vi "Main.vi"() -> ()   [LabVIEW 2026]
doc: "VI TIMESTAMP — DOCUMENTATION\n============================\nInstitut Fresnel | USB-6353 | CTR3 | PFI7 | 100 MHz | LabVIEW 2025\n\n\nOBJECTIF\n--------\nEnregistrer le timestamp absolu de chaque trigger caméra avec une\nprécision hardware de 10 ns. Résultat écrit dans un fichier CSV,\nécrasé à chaque nouvelle acquisition.\n\n\nPRINCIPE\n--------\nCTR3 compte les ticks de l'horloge interne 100 MHz. Le signal trigger\n(P0.4, rebouclé sur PFI7) est l'horloge d'échantillonnage : à chaque\nflanc montant, CTR3 capture la valeur courante du compteur.\n\n T_absolu = T0 + (ticks + offset_rollover) / 100 000 000\n\nT0 = heure système au démarrage (Get Date/Time In Seconds).\noffset_rollover = compensation du débordement 32 bits (rollover ~42.9 s).\n\n\nMACHINE À ÉTATS\n---------------\nIDLE ? INIT ? START ? RUNNING ? WRITE ? STOP ? IDLE\n\n IDLE : attente bouton Start, lecture N (nb frames)\n INIT : création tâche CTR3, config timing PFI7, ouverture CSV, T0\n START : DAQmx Start Task — doit précéder les tâches DO/AO du VI principal\n RUNNING : DAQmx Read non-bloquant (timeout 0.01 s) — boucle sur lui-même\n WRITE : calcul timestamp, gestion rollover, écriture ligne CSV\n STOP : Stop Task, Clear Task, Close File, reset SR\n\n\nGESTION ROLLOVER (dans WRITE)\n------------------------------\n Si ticks < ticks_prev ? offset += 4 294 967 296\n ticks_prev ? ticks (valeur brute, sans offset)\n\n\nSHIFT REGISTERS\n---------------\n état Enum État courant\n task ref DAQmx Task Référence CTR3\n file ref File Refnum Fichier CSV ouvert\n T0 Timestamp Heure au Start\n ticks DBL Valeur DAQmx Read\n ticks_prev DBL (init 0) Ticks de la frame précédente\n offset DBL (init 0) Cumul rollovers × 2^32\n frame_i I32 (init 0) Index frame courante\n\n\nFORMAT CSV\n----------\n frame_index I32 Index frame (0-indexé)\n timestamp_iso String Ex : 2026-03-09T11:13:54.223 (ISO 8601)\n timestamp_unix DBL Ex : 3855896034.224 (secondes depuis 01/01/1904)\n\nConversion Python :\n df['datetime'] = pd.to_datetime(df['timestamp_unix'] - 2082844800, unit='s')\n\n\nVALIDATION\n----------\n 20.9 Hz jitter 358 µs (vient du générateur NI-MAX, pas du VI) ?\n 0.1 Hz 2 rollovers détectés et compensés, monotonie OK ?"
uses:
  controls/State.ctl
  <vilib>/DAQmx/read.llb/DAQmx Read (Counter DBL 1Chan 1Samp).vi
  <vilib>/DAQmx/create/channels.llb/DAQmx Create Channel (CI-Count Edges).vi
  <vilib>/DAQmx/configure/timing.llb/DAQmx Timing (Sample Clock).vi
  <vilib>/DAQmx/miscellaneous.llb/DAQmx Fill In Error Info.vi
  <vilib>/Utility/file.llb/Write Delimited Spreadsheet (DBL).vi
  <resource>/objmgr/daqmx.rc
  <userlib>/_OpenG.lib/error/error.llb/openg_error.lvlib
panel:
  in  "file path (dialog if empty)":path=path "C:/Users/spinning polar/Desktop/TRASH/Ticks.csv"
  out "output array":dbl[](array[numeric])
  out "x >= y?":bool
  out "frame_i":i32
  in  "file path":path=path "C:/Users/spinning polar/Desktop/TRASH/Timestamp.csv"
  in  "samples per channel":i32=10 caption="échantillons par voie"
  in  "Stop":bool
  in  "Start":bool
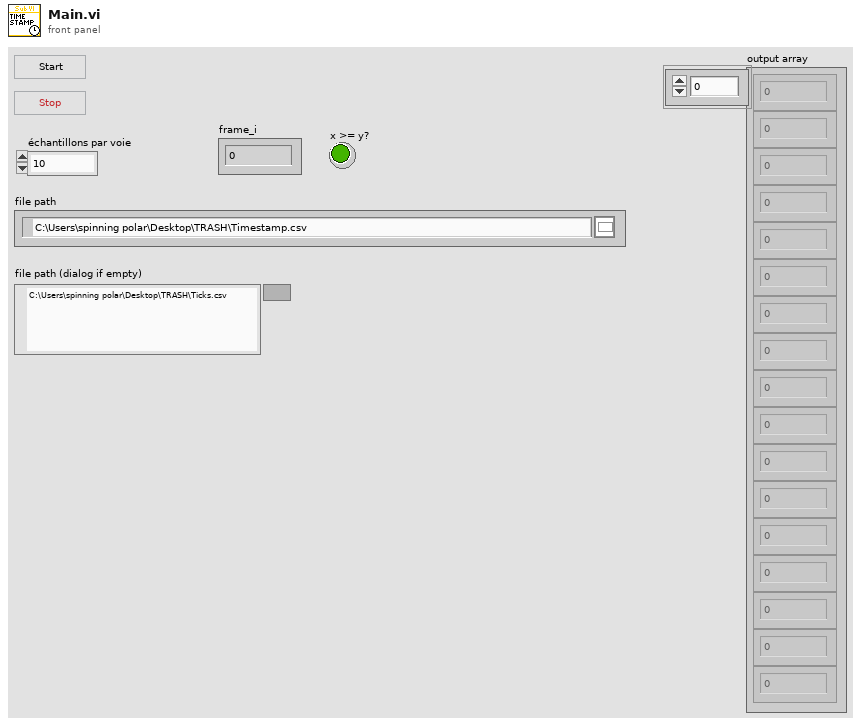
[diagram p1: front panel]
types:
  T1 = typedef "State.ctl" = enum16{"IDLE", "INIT", "START", "RUNNING", "WRITE", "STOP"}
  T2 = enum16{"open", "replace", "create", "open or create", "replace or create", "replace or create with confirmation"}
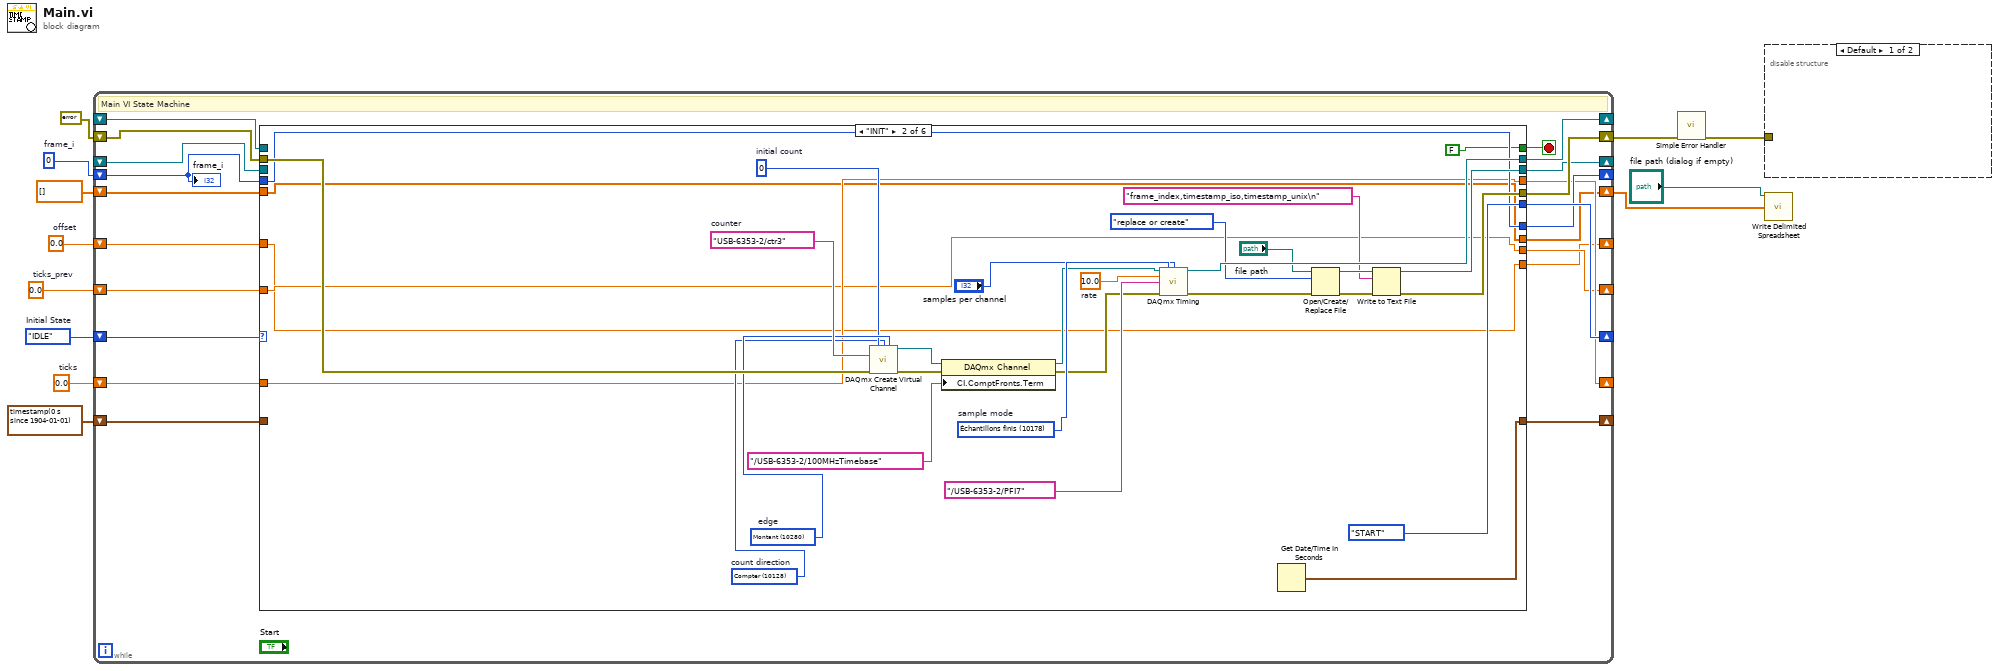
[diagram p0: block diagram]
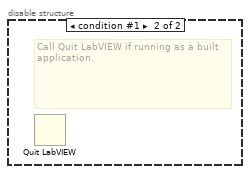
[diagram p2: hidden frame]
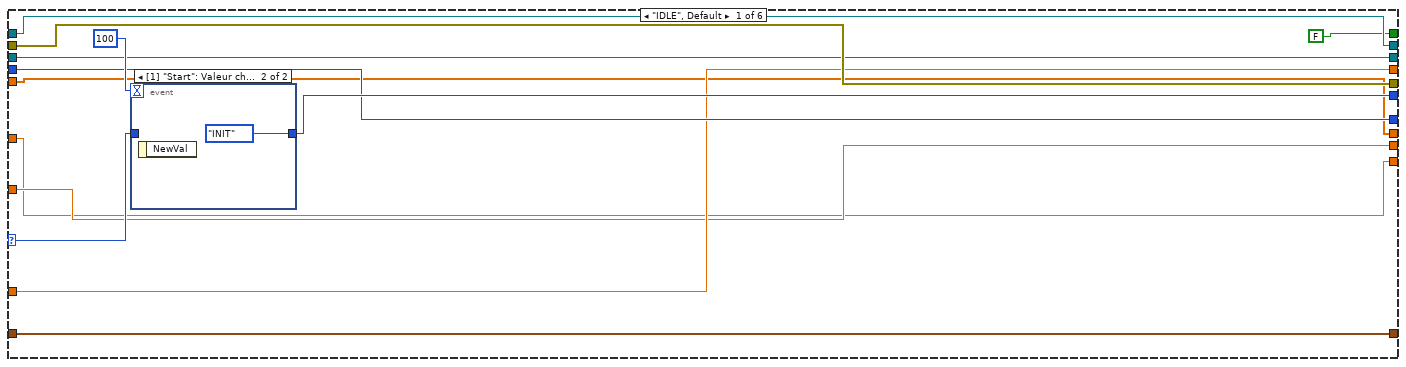
[diagram p3: hidden frame]
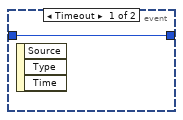
[diagram p4: hidden frame]
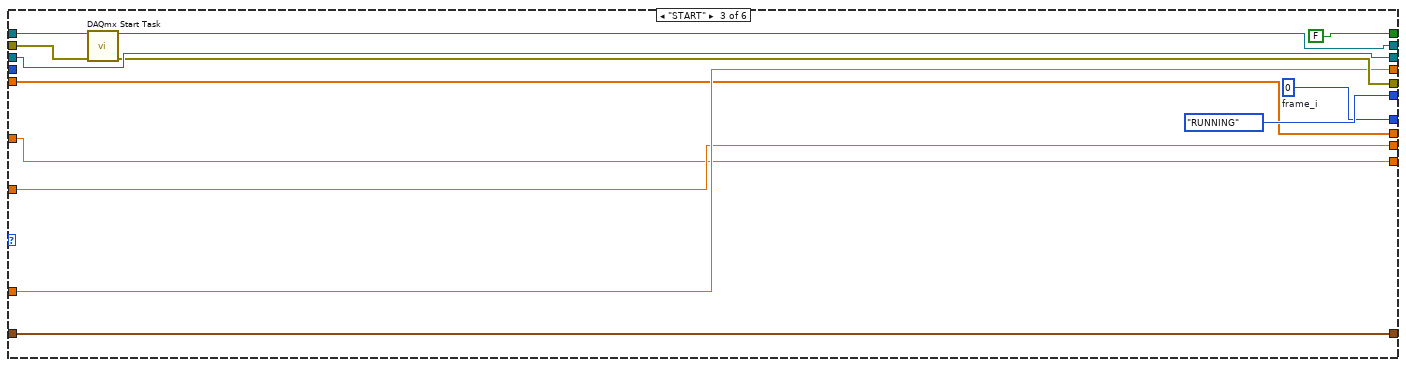
[diagram p5: hidden frame]
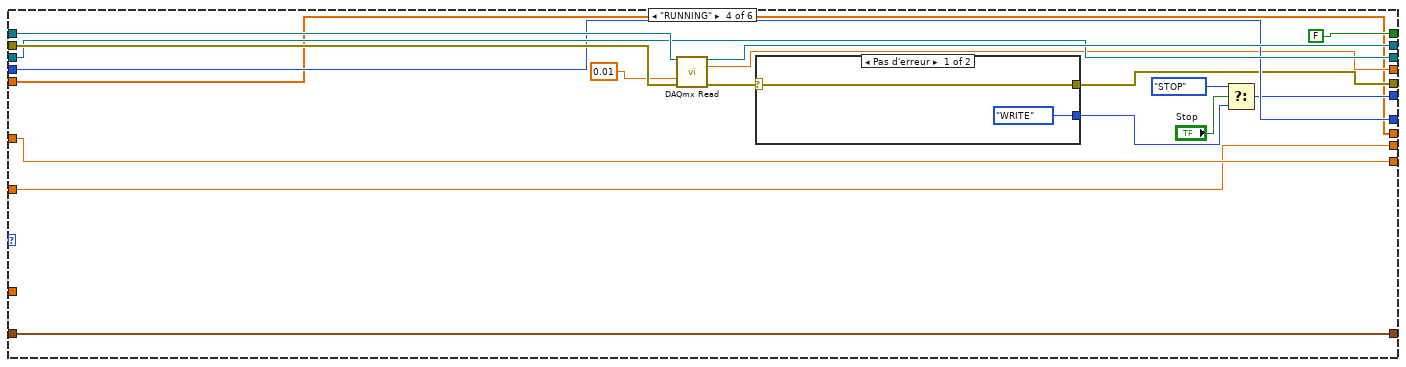
[diagram p6: hidden frame]
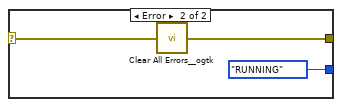
[diagram p7: hidden frame]
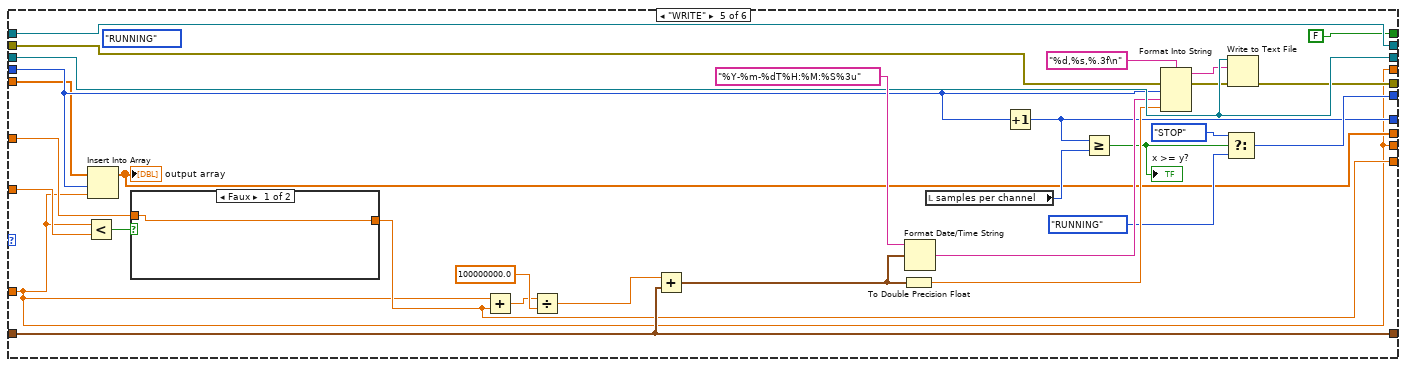
[diagram p8: hidden frame]
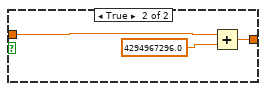
[diagram p9: hidden frame]
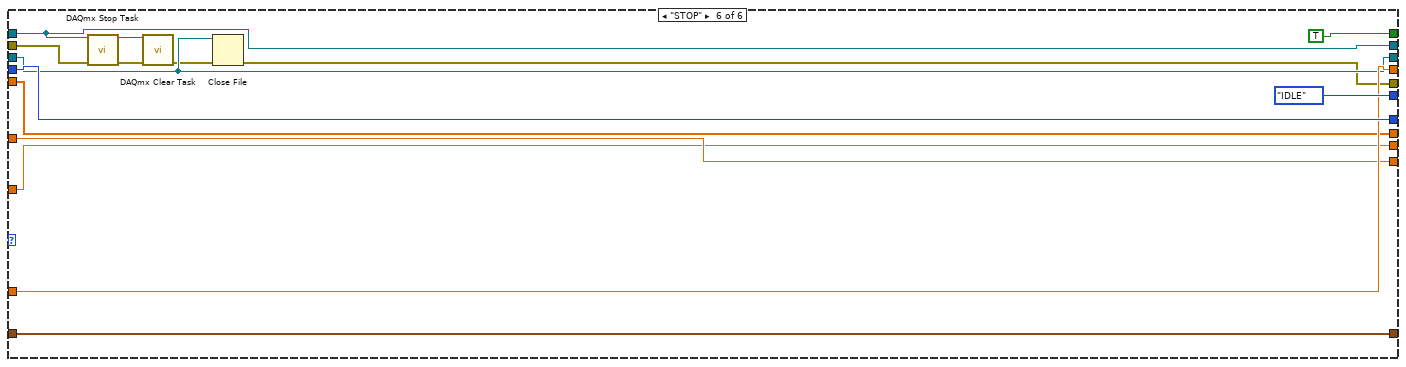
[diagram p10: hidden frame]
diagram:
  w5 = 0.0  # offset
  w4 = 0.0  # ticks_prev
  w7 = 0.0  # ticks
  w8 = 0  # frame_i
  w12 = State."IDLE"  # Initial State
  n1 = while {
    shift-right: [w32] -> _
    shift-left: w12 -> [w33]
    shift-right: [w30] -> w10
    shift-left: errorcluster {"status"=FALSE, "code"=0, "source"=""} ("error constant") -> [w31]
    shift-right: [w29] -> _
    shift-left: _ -> [w28]
    shift-right: [w27] -> _
    shift-left: timestamp(0 s since 1904-01-01) ("seconds since 1Jan1904") -> [w26]
    shift-right: [w25] -> _
    shift-left: _ -> [w24]
    shift-right: [w23] -> _
    shift-left: w8 -> [w22]
    shift-right: [w20] -> _
    shift-left: w7 -> [w19]
    shift-right: [w16] -> _
    shift-left: w5 -> [w15]
    shift-right: [w18] -> _
    shift-left: w4 -> [w17]
    shift-right: [w14] -> w2
    shift-left: dbl[] [] -> [w13]
    stop <- w21 stop-if-true
    # "Main VI State Machine"
    n2 = case shown="\"INIT\"" w33 {
      selector: w33 -> [w44 _ _ _ _ _]
      tunnel: [w45 State."START" ("Initial State") State."RUNNING" ("Initial State") w97 w128 State."IDLE" ("Initial State")] -> w32
      tunnel: w31 -> [w42 w79 w88 w109 w139 w155]
      tunnel: [w42 w66 w85 w101 w135 w153] -> w30
      tunnel: [w43 w73 w86 w108 w145 w158] -> w29
      tunnel: w28 -> [w43 _ w89 w110 w145 w158]
      tunnel: [w41 w70 w91 w105 w142 w162] -> w27
      tunnel: w26 -> [w41 _ w91 w105 w142 w162]
      tunnel: [w40 w64 w92 w107 w138 w156] -> w25
      tunnel: w24 -> [w40 _ w92 w107 w138 w156]
      tunnel: [w39 w54 w87 w106 w122 w163] -> w23
      tunnel: w22 -> [w39 w54 _ w106 w121 w163]
      tunnel: [FALSE ("Stop") FALSE ("Stop") FALSE ("Stop") FALSE ("Stop") FALSE ("Stop") TRUE ("Stop")] -> w21
      tunnel: [w37 w52 w83 w103 w116 w160] -> w20
      tunnel: w19 -> [w37 w52 w83 _ w116 w160]
      tunnel: [w36 w51 w82 w94 w116 w151] -> w18
      tunnel: w17 -> [w36 w51 w82 w94 w125 w151]
      tunnel: [w35 w50 w81 w95 w117 w152] -> w16
      tunnel: w15 -> [w35 w50 w81 w95 w123 w152]
      tunnel: [w34 w49 w80 w93 w120 w150] -> w14
      tunnel: w13 -> [w34 w49 w80 w93 w119 w150]
      frame "IDLE", Default {
        n3 = event shown="[1] \"Start\": Valeur changée" {
          selector: _ -> [_ _]
          dyn-events: _ -> [_ _]
          timeout: 100 -> [_ _]
          tunnel: [w47 State."INIT" ("Initial State")] -> w45
          tunnel: w44 -> [w47 _]
          event Timeout {
            n4 = event-data() -> ()  [unwired: 1 in, 3 out]
          }
          event "Start": Value Change {
            n5 = event-data() -> ()  [unwired: 1 in, 1 out]
          }
        }
      }
      frame "INIT" {
        w60 = 10.0  # rate
        w72 = 10178 items=["Échantillons finis"=10178, "Échantillons continus"=10123, "Point par point avec cadencement matériel"=12522]  # sample mode
        w74 = 10128 items=["Compter"=10128, "Compter à rebours"=10124, "Contrôlé de manière externe"=10326]  # count direction
        w75 = u32 0  # initial count
        w76 = 10280 items=["Montant"=10280, "Descendant"=10171]  # edge
        w77 = tag "USB-6353-2/ctr3"  # counter
        n6 = call-poly <vilib>:"DAQmx Create Virtual Channel.vi"("initial count"=w75, "count direction"=w74, "edge"=w76, "counter"=w77, "error in"=w79) -> ("task out"=w58:refnum<k21>, "error out"=w59:errorcluster)  [unwired: 9 in]
        n7 = property class="DAQmx Channel"(reference=w58, error in=w59, "CI.ComptFronts.Term"=tag "/USB-6353-2/100MHzTimebase") -> (reference out=w57:refnum<k21>, error out=w56:errorcluster)
        n8 = call-poly <vilib>:"DAQmx Timing.vi"("task/channels in"=w57, "sample mode"=w72, "samples per channel"="samples per channel", "rate"=w60, "source"=tag "/USB-6353-2/PFI7", "error in"=w56) -> ("task out"=w73:refnum<k21>, "error out"=w69:errorcluster)  [unwired: 8 in]
        n9 = Get Date/Time In Seconds() -> (seconds since 1Jan1904=w70:timestamp)
        n10 = Open/Create/Replace File(file path (use dialog)="file path", error in=w69, operation (0:open)=T2."replace or create") -> (refnum out=w65:refnum<file>, error out=w67:errorcluster)  [unwired: 3 in, 1 out]
        n11 = Write to Text File(file (use dialog)=w65, text="frame_index,timestamp_iso,timestamp_unix\n", error in=w67) -> (refnum out=w64:refnum<file>, error out=w66:errorcluster)  [unwired: 1 in, 1 out]
      }
      frame "START" {
        w87 = 0  # frame_i
        n12 = call <vilib>:"DAQmx Start Task.vi"("task/channels in"=w89, "error in"=w88) -> ("task out"=w86:refnum<k21>, "error out"=w85:errorcluster)  [unwired: 12 in]
      }
      frame "RUNNING" {
        n13 = call-poly <vilib>:"DAQmx Read.vi"("task/channels in"=w110, "timeout"=0.01, "error in"=w109) -> ("task out"=w108:refnum<k21>, "data"=w103:dbl, "error out"=w102:errorcluster)  [unwired: 10 in]
        n14 = case shown="Pas d'erreur" w102 {
          selector: w102 -> [w111 w114]
          tunnel: [State."WRITE" ("Initial State") State."RUNNING" ("Initial State")] -> w99
          tunnel: [w111 w113] -> w101
          frame No Error {
          }
          frame Error {
            n15 = call <userlib>:"Clear All Errors__ogtk.vi"("Error In"=w114) -> ("Error Out"=w113:errorcluster)  [unwired: 3 in]
          }
        }
        n16 = Select(t=State."STOP" ("Initial State"), s="Stop", f=w99) -> (s? t:f=w97:T1)
      }
      frame "WRITE" {
        (unwired) State."RUNNING" ("Initial State")
        n17 = Less?(x=w116, y=w125) -> (x < y?=w124:bool)
        n18 = Insert Into Array(array=w119, index=w121, new element=w116) -> (w120:dbl[])
        "output array" <- w120
        n19 = case shown="Faux" w124 {
          tunnel: w123 -> [w146 w148]
          tunnel: [w146 w147] -> w117
          frame False {
          }
          frame True {
            n20 = Add(x=w148, y=4294967296.0) -> (x+y=w147:dbl)
          }
        }
        n21 = Add(x=w116, y=w117) -> (x+y=w118:dbl)
        n22 = Divide(x=w118, y=100000000.0) -> (x/y=w143:dbl)
        n23 = Add(x=w143, y=w142) -> (x+y=w133:timestamp)
        n24 = To Double Precision Float(number=w133) -> (double precision float=w132:dbl)
        n25 = Format Date/Time String(time format string (%c)="%Y-%m-%dT%H:%M:%S%3u", seconds (now)=w133) -> (date/time string=w136:string)  [unwired: 1 in]
        n26 = local read "samples per channel"() -> (w131:i32)
        n27 = Increment(x=w121) -> (x+1=w122:i32)
        n28 = Greater Or Equal?(x=w122, y=w131) -> (x >= y?=w127:bool)
        "x >= y?" <- w127
        n29 = Format Into String(format string="%d,%s,%.3f\n", error in=w139, w121, w136, w132) -> (resulting string=w134:string, error out=w137:errorcluster)  [unwired: 1 in]
        n30 = Select(t=State."STOP" ("Initial State"), s=w127, f=State."RUNNING" ("Initial State")) -> (s? t:f=w128:T1)
        n31 = Write to Text File(file (use dialog)=w138, text=w134, error in=w137) -> (error out=w135:errorcluster)  [unwired: 1 in, 2 out]
      }
      frame "STOP" {
        n32 = call <vilib>:"DAQmx Stop Task.vi"("task/channels in"=w158, "error in"=w155) -> ("task out"=w159:refnum<k21>, "error out"=w157:errorcluster)  [unwired: 12 in]
        n33 = call <vilib>:"DAQmx Clear Task.vi"("task in"=w159, "error in"=w157) -> ("error out"=w154:errorcluster)  [unwired: 13 in]
        n34 = Close File(refnum=w156, error in=w154) -> (error out=w153:errorcluster)  [unwired: 1 out]
      }
    }
    "frame_i" <- w22
  }
  n35 = call <vilib>:"Simple Error Handler.vi"("error in (no error)"=w10) -> ("error out"=w9:errorcluster)  [unwired: 4 in, 4 out]
  n36 = disable-structure shown="Default" {
    disable-tunnel: w9 -> [_ _]
    frame condition #0 (active) {
    }
    frame condition #1 {
      # "Call Quit LabVIEW if running as a built application."
      n37 = Quit LabVIEW() -> ()  [unwired: 1 in]
    }
  }
  n38 = call-poly <vilib>:"Write Delimited Spreadsheet.vi"("file path (dialog if empty)"="file path (dialog if empty)", "1D data"=w2) -> ()  [unwired: 12 in, 2 out]
